vi "Read Plot Area Size.vi"(9 "GraphChart in":refnum<class "GraphChart.lvclass">) -> (3 "GraphChart out":refnum<class "GraphChart.lvclass">, 4 "Plot Area Size":cluster{"Width":u32, "Height":u32})   [LabVIEW 2014, in "GraphChart.lvclass"]
uses:
  GraphChart.lvclass
  GraphChart.lvclass/GraphChart.ctl
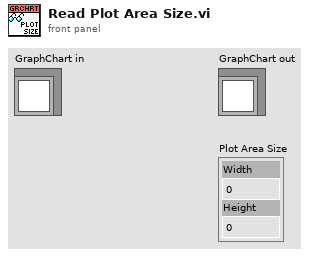
[diagram p1: front panel]
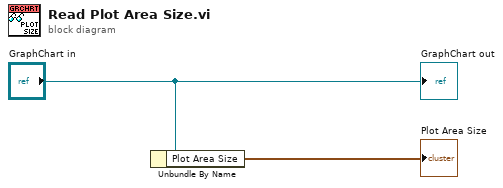
[diagram p0: block diagram]
diagram:
  n1 = Unbundle By Name("GraphChart in") -> ("Plot Area Size"=→"Plot Area Size":cluster{"Width":u32, "Height":u32})
  "GraphChart out" <- "GraphChart in"
